vi "Read Count.vi"(11 "CI Serializer in":refnum<class "CI Serializer.lvclass">) -> (2 "Count":i32)   [LabVIEW 2014, in "CI Serializer.lvclass"]
uses:
  CI Serializer.lvclass
  CI Serializer.lvclass/CI Serializer.ctl
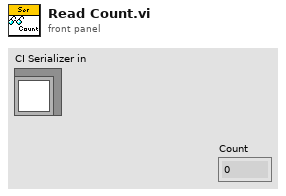
[diagram p1: front panel]
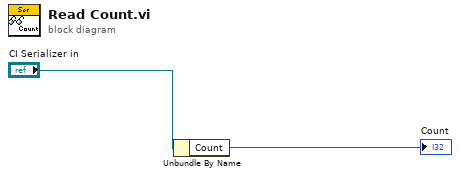
[diagram p0: block diagram]
diagram:
  n1 = Unbundle By Name("CI Serializer in") -> ("Count"=→"Count":i32)
